vi "Untitled 199.vi"() -> ()   [LabVIEW 2017]
panel:
  in  "Montant":dbl
  in  "stop":bool
  in  "10":bool
  in  "5":bool
  out "Boolean":bool
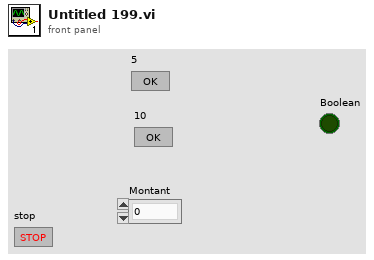
[diagram p1: front panel]
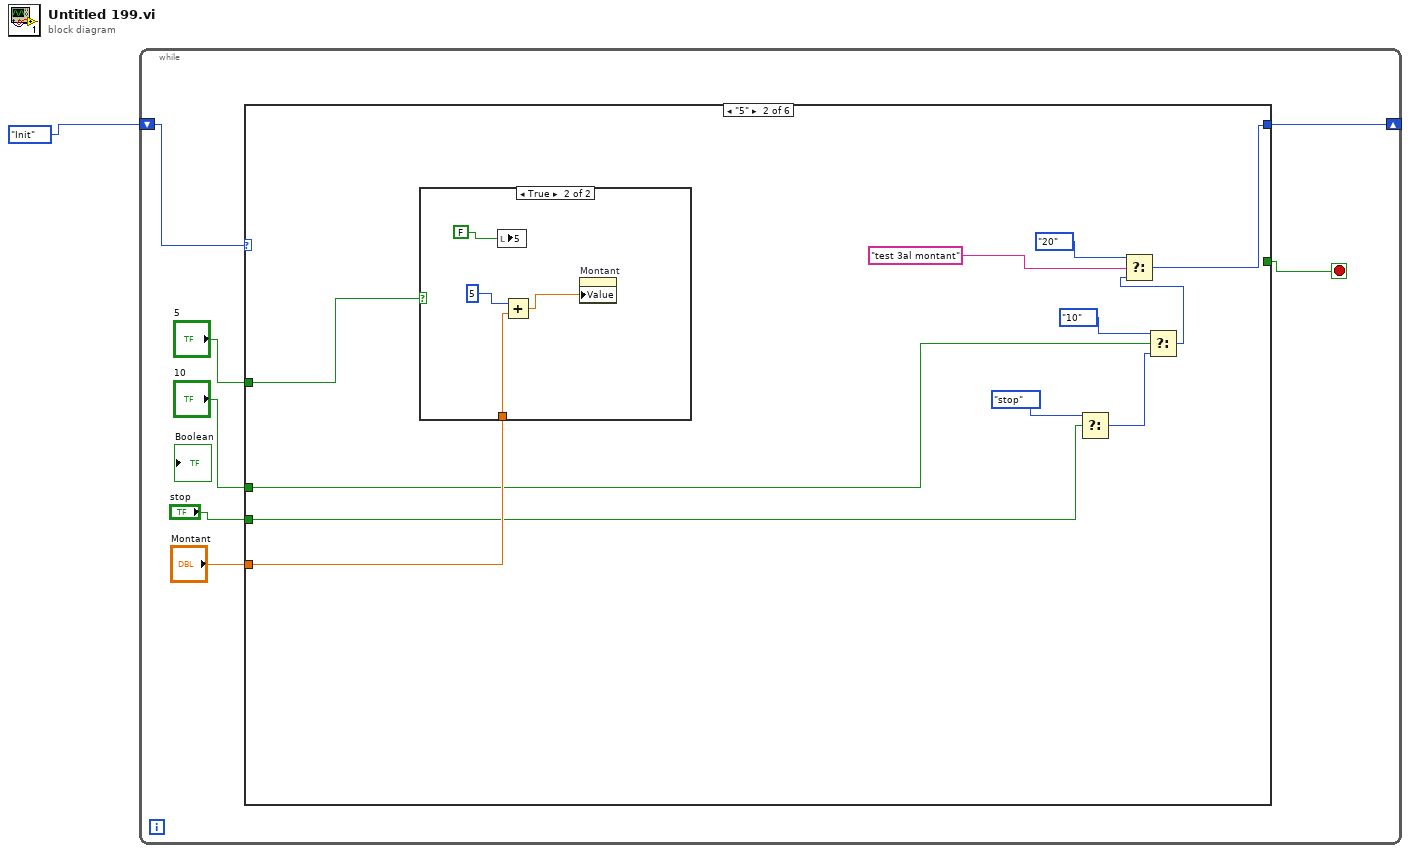
[diagram p0: block diagram]
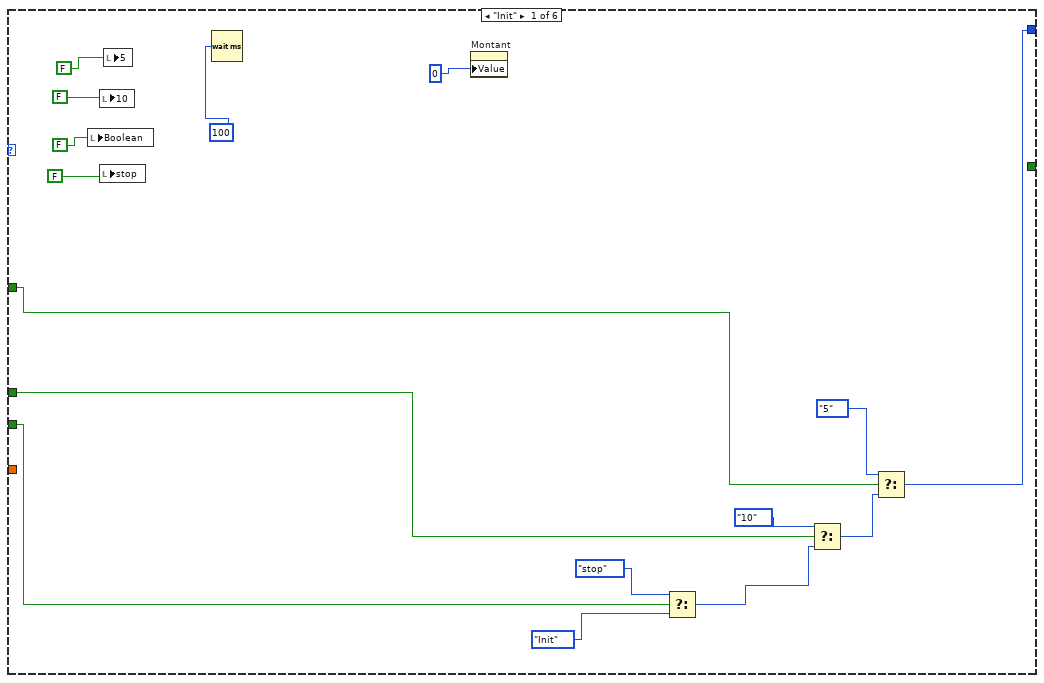
[diagram p2: hidden frame]
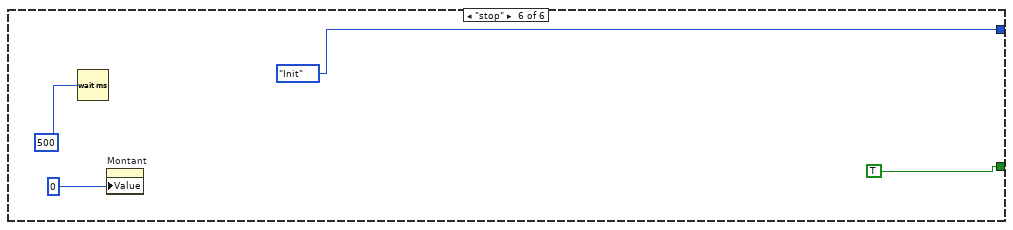
[diagram p7: hidden frame]
diagram:
  n1 = while {
    shift-right: [w8] -> _
    shift-left: enum16{"Init", "5", "10", "15", "20", "stop"}."Init" -> [w7]
    stop <- w2 stop-if-true
    n2 = case shown="\"5\"" w7 {
      tunnel: [w9 w34 _ _ _ enum16{"Init", "5", "10", "15", "20", "stop"}."Init"] -> w8
      tunnel: "5" -> [w17 w26 _ _ _ _]
      tunnel: "10" -> [w10 w28 _ _ _ _]
      tunnel: "Montant" -> [_ w35 _ _ _ _]
      tunnel: "stop" -> [w11 w27 _ _ _ _]
      tunnel: [_ _ _ _ _ TRUE] -> w2
      frame "Init" {
        n3 = local write "Boolean"(FALSE) -> ()
        n4 = local write "10"(FALSE) -> ()
        n5 = local write "stop"(FALSE) -> ()
        n6 = local write "5"(FALSE) -> ()
        n7 = Wait (ms)(milliseconds to wait=100) -> ()  [unwired: 1 out]
        n8 = property on="Montant" class="DigNum (strict)"("Value"=0) -> ()  [unwired: 2 in, 2 out]
        n9 = Select(t=enum16{"Init", "5", "10", "15", "20", "stop"}."stop", s=w11, f=enum16{"Init", "5", "10", "15", "20", "stop"}."Init") -> (s? t:f=w14:enum16{"Init", "5", "10", "15", "20", "stop"})
        n10 = Select(t=enum16{"Init", "5", "10", "15", "20", "stop"}."10", s=w10, f=w14) -> (s? t:f=w16:enum16{"Init", "5", "10", "15", "20", "stop"})
        n11 = Select(t=enum16{"Init", "5", "10", "15", "20", "stop"}."5", s=w17, f=w16) -> (s? t:f=w9:enum16{"Init", "5", "10", "15", "20", "stop"})
      }
      frame "5" {
        n12 = case shown="True" w26 {
          tunnel: w35 -> [_ w36]
          frame False {
          }
          frame True {
            n13 = local write "5"(FALSE) -> ()
            n14 = Add(x=5, y=w36) -> (x+y=w37:dbl)
            n15 = property on="Montant" class="DigNum (strict)"("Value"=w37) -> ()  [unwired: 2 in, 2 out]
          }
        }
        n16 = Select(t=enum16{"Init", "5", "10", "15", "20", "stop"}."stop", s=w27) -> (s? t:f=w30:enum16{"Init", "5", "10", "15", "20", "stop"})  [unwired: 1 in]
        n17 = Select(t=enum16{"Init", "5", "10", "15", "20", "stop"}."10", s=w28, f=w30) -> (s? t:f=w29:enum16{"Init", "5", "10", "15", "20", "stop"})
        n18 = Select(t=enum16{"Init", "5", "10", "15", "20", "stop"}."20", s="test 3al montant", f=w29) -> (s? t:f=w34:enum16{"Init", "5", "10", "15", "20", "stop"})
      }
      frame "10" {
      }
      frame "15" {
      }
      frame "20" {
      }
      frame "stop" {
        n19 = Wait (ms)(milliseconds to wait=500) -> ()  [unwired: 1 out]
        n20 = property on="Montant" class="DigNum (strict)"("Value"=0) -> ()  [unwired: 2 in, 2 out]
      }
    }
  }
